vi "_FPGA Read Counter.vi"(3 "error in (no error)":errorcluster) -> (0 "error out":errorcluster, 1 "size(s)":u32, 2 "Data":i32[](array[numeric]))   [LabVIEW 2012]
uses:
  _RT Global.vi
  <vilib>/Utility/error.llb/Error Cluster From Error Code.vi
  <vilib>/rvi/errors/niLvFpgaAdjustHostInterfaceError.vi
  <vilib>/rvi/interface/nirviMethod/nirviMethod.xnode
  FPGA Bitfiles/FPGA9602.lvbitx
  <vilib>/FPGAPlugInAG/sbRIO-9602/niLvFpga_ReadFifo_sbRIO-9602.vi
  <vilib>/rvi/errors/niLvFpgaMergeErrorWithErrorCode.vi
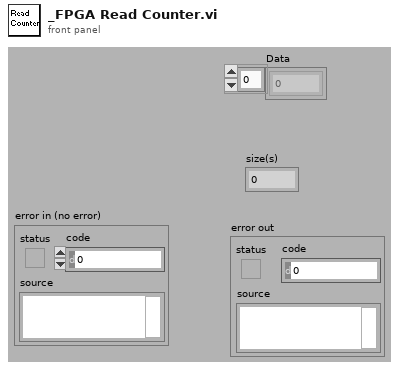
[diagram p1: front panel]
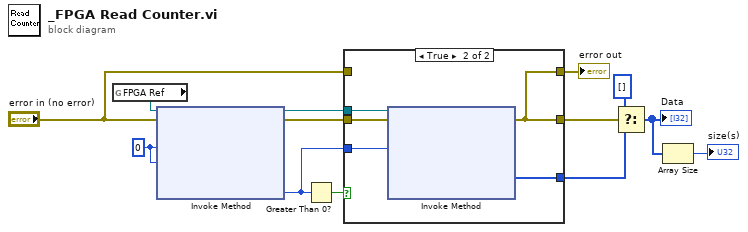
[diagram p0: block diagram]
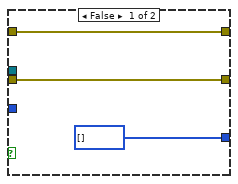
[diagram p2: hidden frame]
diagram:
  w8 = u32 0 ("Number of Elements")
  n1 = global read "_RT Global.vi" "FPGA Ref"() -> (w1:refnum<k20>)
  n2 = xnode "Invoke Method"("FPGA VI Reference In"=w1, "error in"="error in (no error)", "Number of Elements"=w8, "Timeout (ms)"=w8) -> ("FPGA VI Reference Out"=w4:refnum<k20>, "error out"=w5:errorcluster, "Elements Remaining"=w6:u32)  [unwired: 1 out]
  n3 = Greater Than 0?(x=w6) -> (x > 0?=w7:bool)
  n4 = case shown="True" w7 {
    tunnel: w4 -> [_ w21]
    tunnel: w5 -> [w16 w20]
    tunnel: w6 -> [_ w19]
    tunnel: [u32[] [] ("Data") w17] -> w12
    tunnel: [w16 w18] -> w13
    tunnel: [w15 w18] -> w3
    tunnel: "error in (no error)" -> [w15 _]
    frame False {
    }
    frame True {
      n5 = xnode "Invoke Method"("FPGA VI Reference In"=w21, "error in"=w20, "Number of Elements"=w19) -> ("error out"=w18:errorcluster, "Data"=w17:u32[])  [unwired: 1 in, 2 out]
    }
  }
  "error out" <- w3
  n6 = Select(t=u32[] [], s=w13, f=w12) -> (s? t:f=w10:u32[])
  "Data" <- w10
  n7 = Array Size(array=w10) -> (size(s)=→"size(s)":i32)
